vi "XYZ_reset.vi"   [LabVIEW 2023]
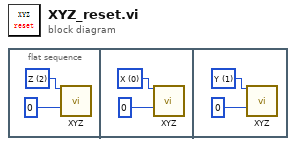
[diagram p0: block diagram]
diagram:
  n1 = flat-sequence {
    frame #0 {
      w2 = u16 2 items=["X", "Y", "Z"] ("AXIS")
      n2 = call "XYZ.vi"("AXIS"=w2, "Set location (mm)"=0) -> ()  [unwired: 9 in, 5 out]
    }
    frame #1 {
      w3 = u16 0 items=["X", "Y", "Z"] ("AXIS")
      n3 = call "XYZ.vi"("AXIS"=w3, "Set location (mm)"=0) -> ()  [unwired: 9 in, 5 out]
    }
    frame #2 {
      w6 = u16 1 items=["X", "Y", "Z"] ("AXIS")
      n4 = call "XYZ.vi"("AXIS"=w6, "Set location (mm)"=0) -> ()  [unwired: 9 in, 5 out]
    }
  }
